vi "Limit_Line_Table.vi"() -> (0 "状态":string, 1 "Limit_ISL":string[][](array[string]), 2 "Limit_VSWR":string[][](array[string]), 3 "Limit_IL":string[][](array[string]))   [LabVIEW 2020]
uses:
  <vilib>/Utility/NIReport.llb/Report Type.ctl
  <vilib>/addons/_office/excel.llb/Excel Get Data ([str]).vi
  <vilib>/Utility/NIReport.llb/Append Text Table to Report (wrap).vi
  <vilib>/Utility/NIReport.llb/NI_report.lvclass
  <vilib>/Utility/NIReport.llb/NI_ReportGenerationCore.lvlib
  <vilib>/Utility/NIReport.llb/Excel/NI_Excel.lvclass
  <vilib>/addons/_office/NI_ReportGenerationToolkit.lvlib
panel:
  in  "插入损耗IL":i32(listbox)
  in  "驻波VSWR":i32(listbox) caption="多列列表框VSWR"
  in  "隔离度ISL":i32(listbox) caption="多列列表框VSWR"
  in  "清空":bool
  in  "导入":bool
  in  "保存":bool
  in  "取消":bool
  in  "确定":bool
  # "Limit Line"
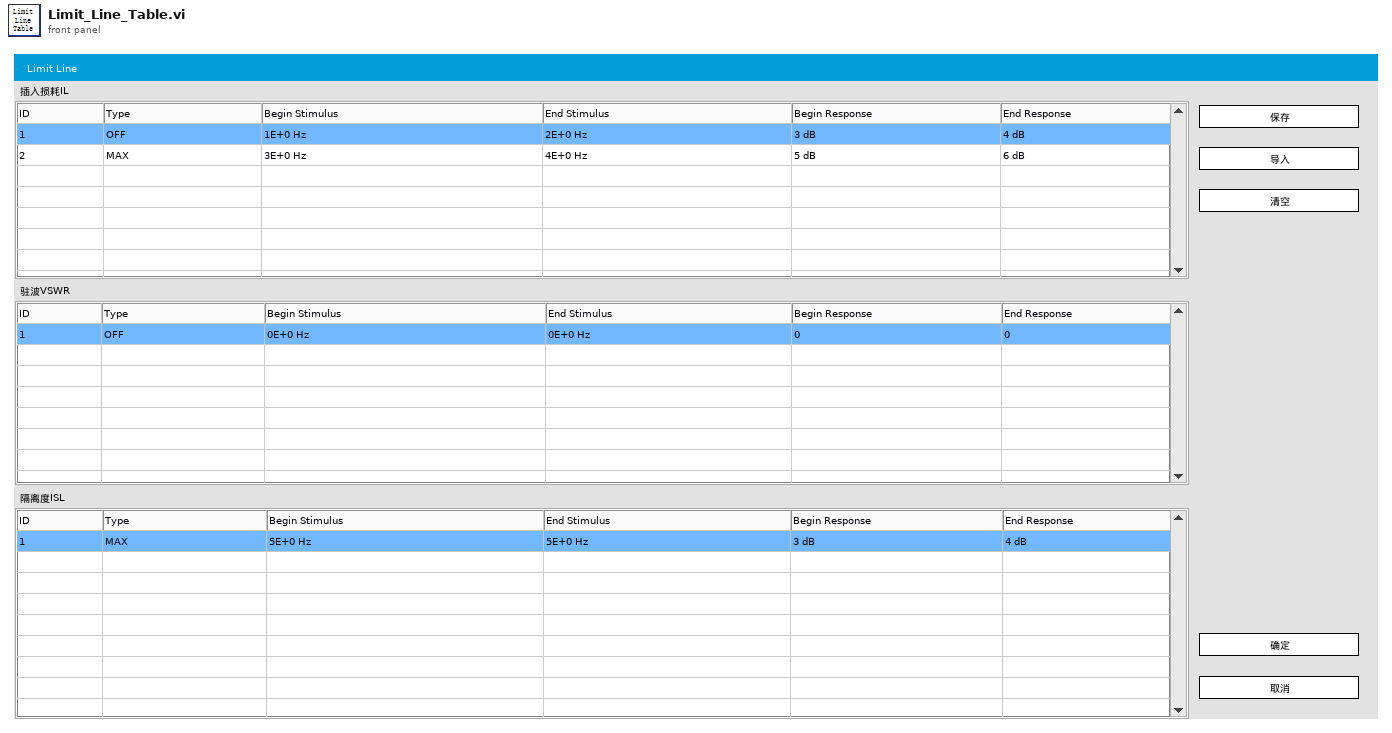
[diagram p1: front panel]
types:
  T1 = typedef "NI_ReportGenerationCore.lvlib/Report Type.ctl" = enum16{"HTML", "Word", "Excel"}
  T2 = enum16{"maximized", "minimized", "normal", "no change"}
  T3 = typedef "LVPoint32TypeDef.ctl" = cluster{"Horizontal":i32, "Vertical":i32}
  T4 = typedef "LVRowAndColumnTypeDef.ctl" = cluster{"Row":i32, "Column":i32}
  T5 = enum32{"invalid app kind", "Development System", "Run Time System", "Student Edition", "Embedded LabVIEW", "Evaluation", "Custom"}
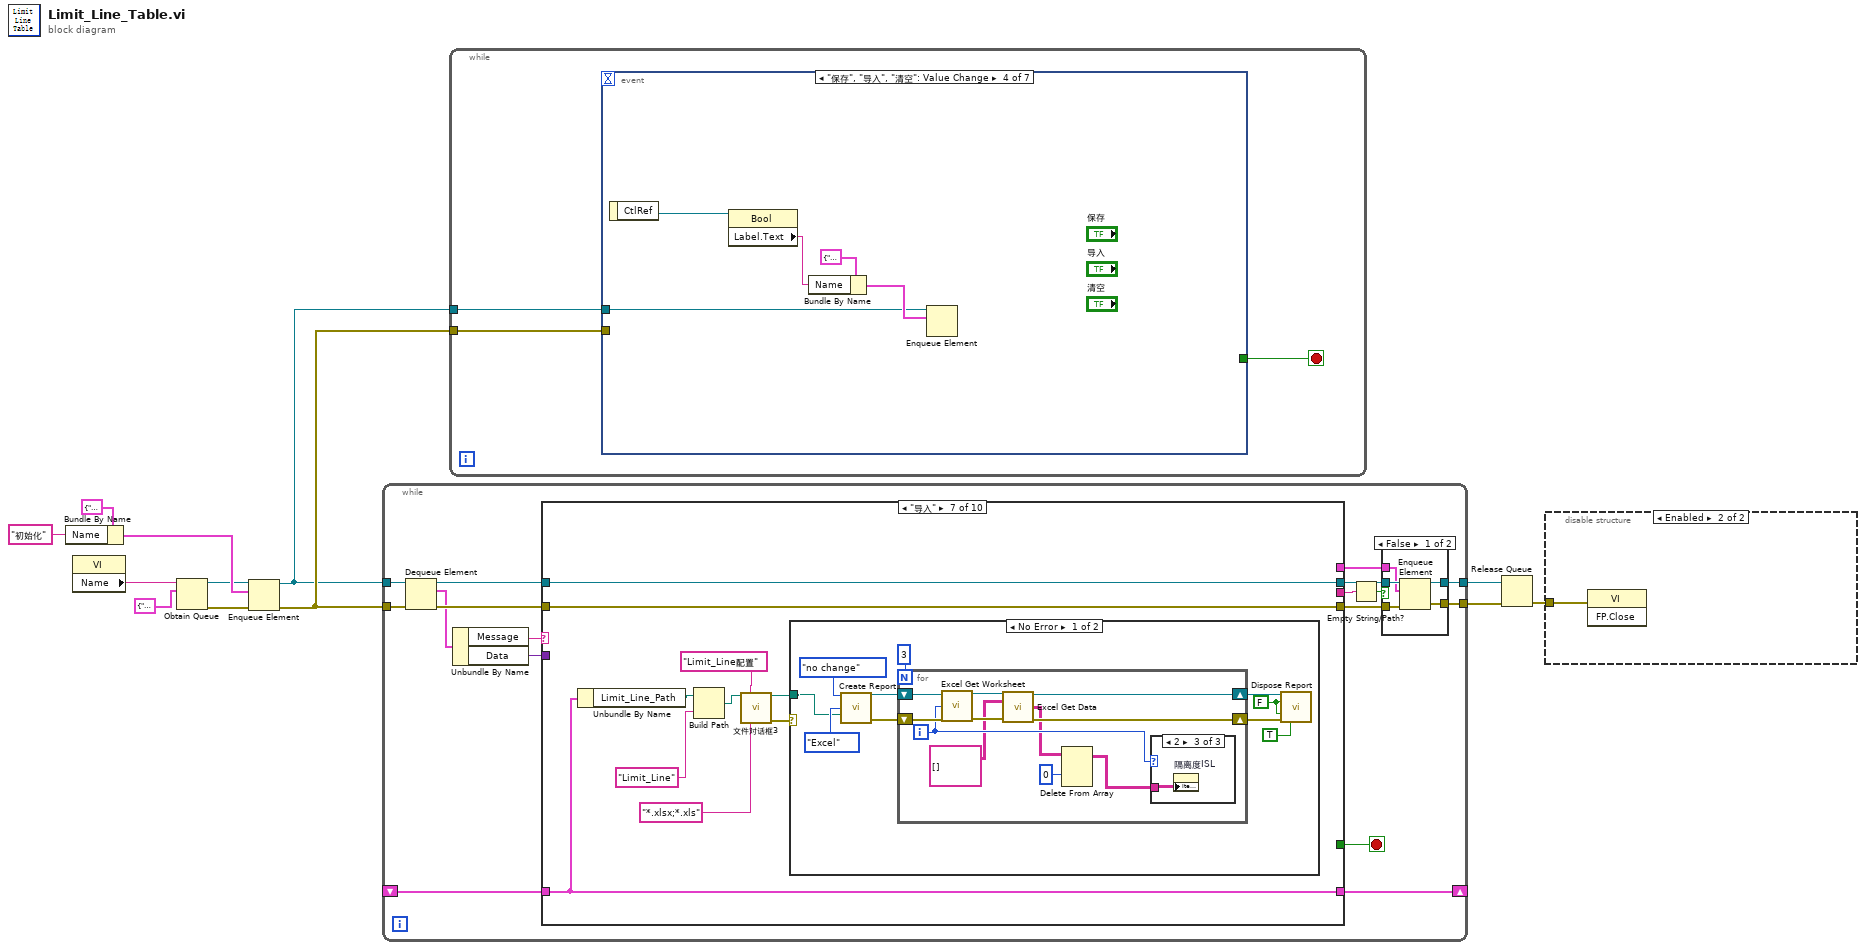
[diagram p0: block diagram]
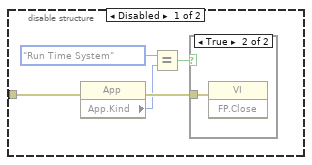
[diagram p2: hidden frame]
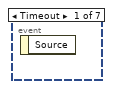
[diagram p4: hidden frame]
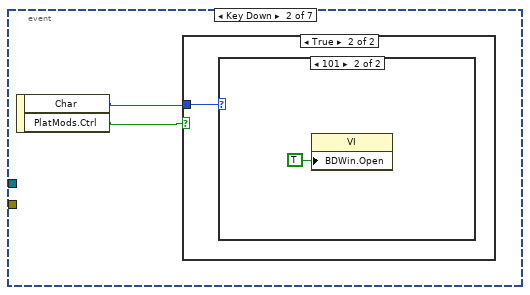
[diagram p5: hidden frame]
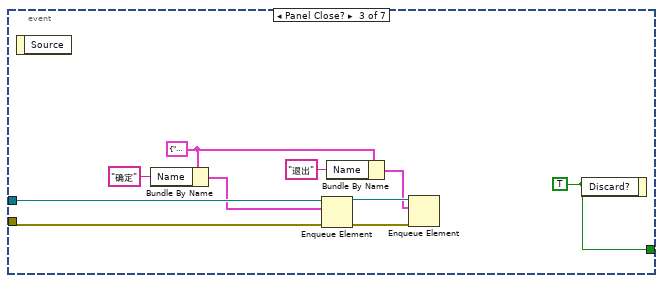
[diagram p8: hidden frame]
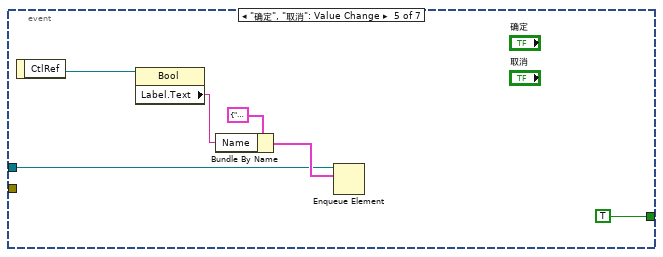
[diagram p9: hidden frame]
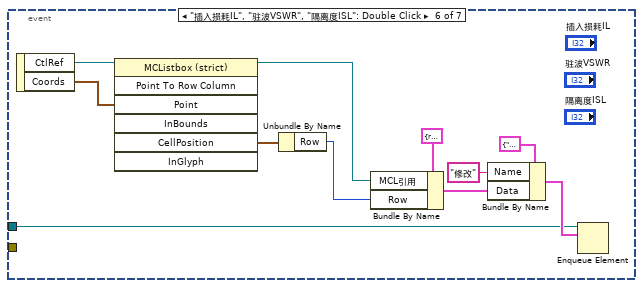
[diagram p10: hidden frame]
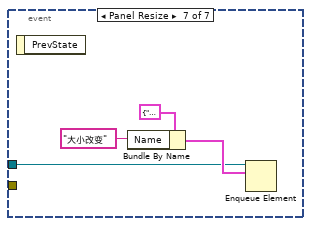
[diagram p11: hidden frame]
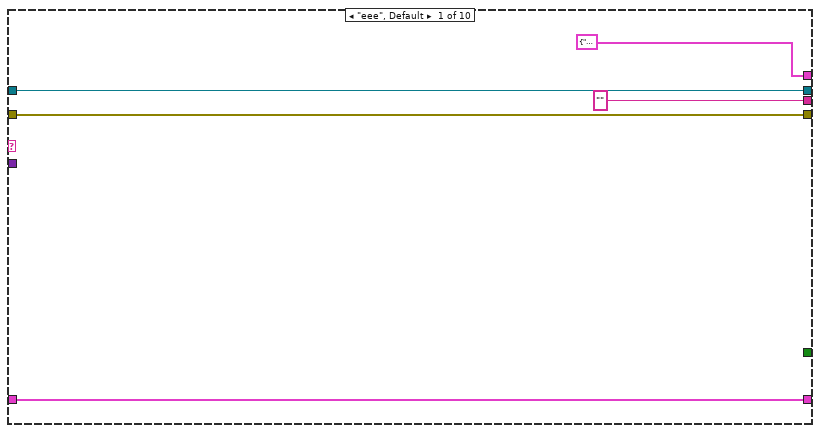
[diagram p13: hidden frame]
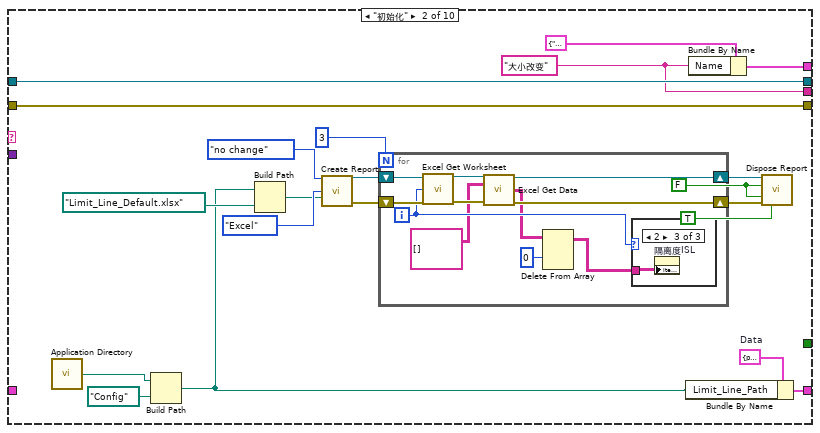
[diagram p14: hidden frame]
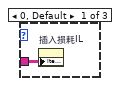
[diagram p15: hidden frame]
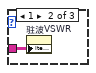
[diagram p16: hidden frame]
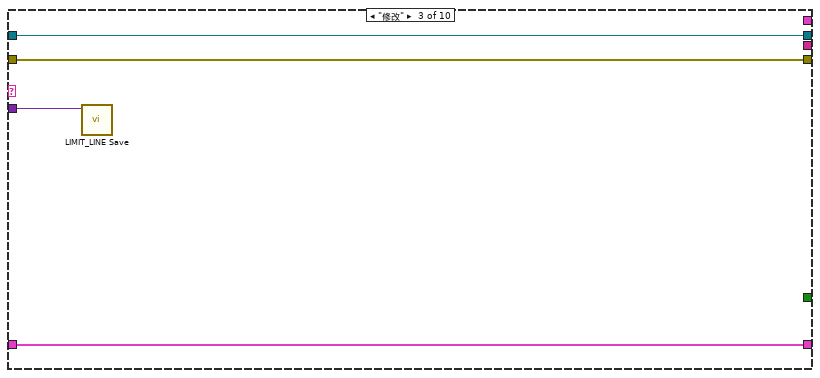
[diagram p17: hidden frame]
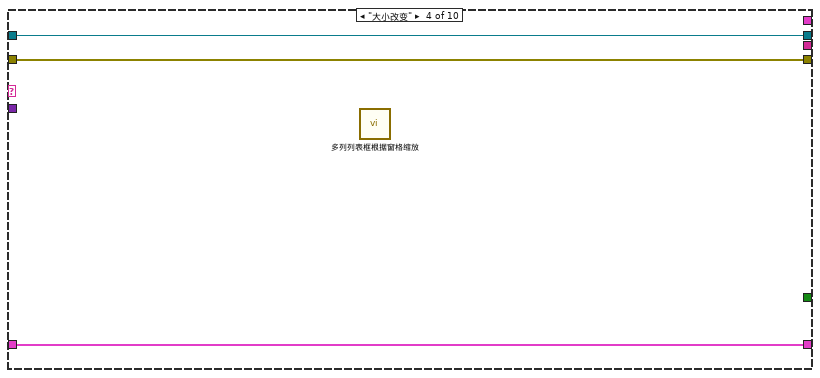
[diagram p18: hidden frame]
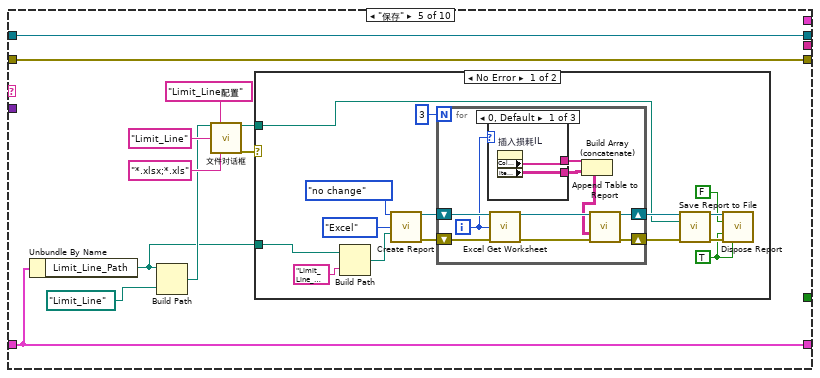
[diagram p19: hidden frame]
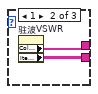
[diagram p20: hidden frame]
diagram:
  n1 = Bundle By Name(cluster=cluster{"Name":string, "Data":variant} {"Name"="", "Data"=variant}, "Name"="初始化") -> (w12:cluster{"Name":string, "Data":variant})
  n2 = property class="VI"() -> ("Name"=w2:string)  [unwired: 2 in, 2 out]
  n3 = Obtain Queue(name (unnamed)=w2, element data type=cluster{"Message":string, "Data":variant} {"Message"="", "Data"=variant}) -> (queue out=w4:refnum<queue>, error out=w3:errorcluster)  [unwired: 3 in, 1 out]
  n4 = Enqueue Element(queue=w4, element=w12, error in (no error)=w3) -> (queue out=w7:refnum<queue>, error out=w8:errorcluster)  [unwired: 1 in, 1 out]
  n5 = while {
    tunnel: w7 -> [w29]
    tunnel: w8 -> [w28]
    tunnel: [w23] -> w5
    tunnel: [w22] -> w6
    shift-right: [w14] -> _
    shift-left: _ -> [w13]
    stop <- w21 stop-if-true
    n6 = Dequeue Element(queue=w29, error in (no error)=w28) -> (queue out=w27:refnum<queue>, element=w17:cluster{"Message":string, "Data":variant}, error out=w24:errorcluster)  [unwired: 1 in, 1 out]
    n7 = Unbundle By Name(w17) -> ("Message"=w16:string, "Data"=w15:variant)
    n8 = case shown="\"导入\"" w16 {
      selector: w16 -> [_ _ _ _ _ _ _ w171 w211 _]
      tunnel: w27 -> [w41 w62 w80 w83 w94 w133 w145 w193 w217 w226]
      tunnel: [w41 w62 w80 w83 w94 w133 w145 w193 w217 w225] -> w26
      tunnel: [w40 w61 w79 w82 w93 w132 w144 w192 w216 w223] -> w25
      tunnel: w24 -> [w40 w61 w79 w82 w93 w132 w144 w192 w216 w224]
      tunnel: [_ _ _ _ _ _ _ _ _ TRUE] -> w21
      tunnel: ["" w57 _ _ _ _ _ w189 w213 _] -> w20
      tunnel: [cluster{"Name":string, "Data":variant} {"Name"="", "Data"=variant} w56 _ _ _ _ _ w190 w215 _] -> w18
      tunnel: w15 -> [_ _ w78 _ _ _ _ _ _ _]
      tunnel: [w37 w54 w77 w81 w87 w126 w142 w170 w210 w219] -> w14
      tunnel: w13 -> [w37 _ w77 w81 w87 w126 w142 w172 w212 w219]
      frame "eee", Default {
      }
      frame "初始化" {
        w48 = FALSE ("wait until printing completed? (T)")
        w55 = cluster{"Limit_Line_Path":path, "状态":string} {"Limit_Line_Path"=path "", "状态"=""}  # Data
        w57 = "大小改变"
        n9 = call <vilib>:"Application Directory.vi"() -> ("Application Directory"=w60:path)
        n10 = Build Path(base path=w60, name or relative path=path "Config" ("名称或相对路径")) -> (appended path=w42:path)
        n11 = Build Path(base path=w42, name or relative path=path "Limit_Line_Default.xlsx" ("名称或相对路径")) -> (appended path=w43:path)
        n12 = call <vilib>:"Create Report.vi"("window state (normal)"=T2."no change", "report type"=Report_Type."Excel", "template (empty)"=w43) -> ("report out"=w53:refnum<class "NI_report.lvclass">, "error out"=w52:errorcluster)  [unwired: 11 in]
        n13 = for {
          N: 3 -> [_]
          shift-right: [w68] -> w50
          shift-left: w53 -> [w71]
          shift-right: [w69] -> w51
          shift-left: w52 -> [w70]
          i -> [w67]
          n14 = call <vilib>:"Excel Get Worksheet.vi"("report in"=w71, "worksheet index (0)"=w67, "error in (no error)"=w70) -> ("report out"=w73:refnum<class "NI_report.lvclass">, "error out"=w72:errorcluster)  [unwired: 11 in]
          n15 = call-poly <vilib>:"Excel Get Data.vi"("report in"=w73, "data type"=string[][] [], "error in (no error)"=w72) -> ("report out"=w68:refnum<class "NI_report.lvclass">, "data"=w65:string[][], "error out"=w69:errorcluster)  [unwired: 10 in]
          n16 = Delete From Array(array=w65, index (row)=0) -> (array with subset deleted=w63:string[][])  [unwired: 2 in, 1 out]
          n17 = case shown="2" w67 {
            tunnel: w63 -> [w74 w75 w76]
            frame 0, Default {
              n18 = property on="插入损耗IL" class="MCListbox (strict)"("ItemNames"=w74) -> ()  [unwired: 2 in, 2 out]
            }
            frame 1 {
              n19 = property on="驻波VSWR" class="MCListbox (strict)"("ItemNames"=w75) -> ()  [unwired: 2 in, 2 out]
            }
            frame 2 {
              n20 = property on="隔离度ISL" class="MCListbox (strict)"("ItemNames"=w76) -> ()  [unwired: 2 in, 2 out]
            }
          }
        }
        n21 = Bundle By Name(cluster=w55, "Limit_Line_Path"=w42) -> (w54:cluster{"Limit_Line_Path":path, "状态":string})
        n22 = Bundle By Name(cluster=cluster{"Name":string, "Data":variant} {"Name"="", "Data"=variant}, "Name"=w57) -> (w56:cluster{"Name":string, "Data":variant})
        n23 = call-dynamic "Dispose Report.vi"("report in"=w50, "wait until printing completed? (T)"=w48, "save changes? (F)"=w48, "error in (no error)"=w51, "close report? (T)"=TRUE ("wait until printing completed? (T)")) -> ()  [unwired: 10 in, 1 out]
      }
      frame "修改" {
        n24 = call "LIMIT_LINE Save.vi"("data"=w78) -> ()  [unwired: 11 in]
      }
      frame "大小改变" {
        n25 = call "多列列表框根据窗格缩放.vi"() -> ()  [unwired: 11 in, 1 out]
      }
      frame "保存" {
        n26 = Unbundle By Name(w87) -> ("Limit_Line_Path"=w84:path)
        n27 = Build Path(base path=w84, name or relative path=path "Limit_Line") -> (appended path=w85:path)
        n28 = call "文件对话框"("start path"=w85, "prompt"="Limit_Line配置" ("default name"), "default name"="Limit_Line", "pattern (all files)"="*.xlsx;*.xls") -> ("selected path"=w92:path, "error out"=w91:errorcluster)  [unwired: 8 in, 2 out]
        n29 = case shown="No Error" w91 {
          tunnel: w92 -> [w98 _]
          tunnel: w84 -> [w95 _]
          frame No Error {
            w103 = TRUE ("save changes? (F)")
            n30 = Build Path(base path=w95, name or relative path="Limit_Line_Template.xlsx") -> (appended path=w96:path)
            n31 = call <vilib>:"Create Report.vi"("window state (normal)"=T2."no change", "report type"=Report_Type."Excel", "template (empty)"=w96) -> ("report out"=w100:refnum<class "NI_report.lvclass">, "error out"=w101:errorcluster)  [unwired: 11 in]
            n32 = for {
              N: 3 -> [_]
              shift-right: [w118] -> w107
              shift-left: w101 -> [w117]
              shift-right: [w119] -> w108
              shift-left: w100 -> [w115]
              i -> [w111]
              n33 = case shown="0, Default" w111 {
                tunnel: [w121 w123 w125] -> w112
                tunnel: [w120 w122 w124] -> w113
                frame 0, Default {
                  n34 = property on="插入损耗IL" class="MCListbox (strict)"() -> ("ColHdrString"=w121:string[], "ItemNames"=w120:string[][])  [unwired: 2 in, 2 out]
                }
                frame 1 {
                  n35 = property on="驻波VSWR" class="MCListbox (strict)"() -> ("ColHdrString"=w123:string[], "ItemNames"=w122:string[][])  [unwired: 2 in, 2 out]
                }
                frame 2 {
                  n36 = property on="隔离度ISL" class="MCListbox (strict)"() -> ("ColHdrString"=w125:string[], "ItemNames"=w124:string[][])  [unwired: 2 in, 2 out]
                }
              }
              n37 = call <vilib>:"Excel Get Worksheet.vi"("report in"=w115, "worksheet index (0)"=w111, "error in (no error)"=w117) -> ("report out"=w114:refnum<class "NI_report.lvclass">, "error out"=w116:errorcluster)  [unwired: 11 in]
              n38 = Build Array (concatenate)(w112, w113) -> (w110:string[][])
              n39 = call-poly <vilib>:"Append Table to Report.vi"("report in"=w114, "text data"=w110, "error in (no error)"=w116) -> ("report out"=w119:refnum<class "NI_report.lvclass">, "error out"=w118:errorcluster)  [unwired: 9 in, 2 out]
            }
            n40 = call-dynamic "Save Report to File.vi"("report in"=w108, "report file path"=w98, "error in (no error)"=w107) -> ("report out"=w106:refnum<class "NI_report.lvclass">, "error out"=w105:errorcluster)  [unwired: 11 in]
            n41 = call-dynamic "Dispose Report.vi"("report in"=w106, "wait until printing completed? (T)"=FALSE, "save changes? (F)"=w103, "error in (no error)"=w105, "close report? (T)"=w103) -> ()  [unwired: 10 in, 1 out]
          }
          frame Error {
          }
        }
      }
      frame "清空" {
        n42 = control-ref of="插入损耗IL"() -> (w131:refnum<vi>)
        n43 = control-ref of="驻波VSWR"() -> (w130:refnum<vi>)
        n44 = control-ref of="隔离度ISL"() -> (w129:refnum<vi>)
        n45 = Build Array(w131, w130, w129) -> (w128:refnum<vi>[])
        n46 = for {
          tunnel: w128 -> [w135] mode=indexing
          tunnel: string[][] [] ("项名") -> [w134]
          n47 = property class="MCListbox (strict)"(reference=w135, "ItemNames"=w134) -> ()  [unwired: 1 in, 2 out]
        }
      }
      frame "导入" {
        n48 = Unbundle By Name(w142) -> ("Limit_Line_Path"=w138:path)
        n49 = Build Path(base path=w138, name or relative path="Limit_Line" ("default name")) -> (appended path=w136:path)
        n50 = call "文件对话框3"("start path"=w136, "prompt"="Limit_Line配置" ("default name"), "pattern (all files)"="*.xlsx;*.xls") -> ("selected path"=w139:path, "error out"=w140:errorcluster)  [unwired: 9 in, 2 out]
        n51 = case shown="No Error" w140 {
          tunnel: w139 -> [w154 _]
          frame No Error {
            w147 = FALSE ("wait until printing completed? (T)")
            n52 = call <vilib>:"Create Report.vi"("window state (normal)"=T2."no change", "report type"=Report_Type."Excel", "template (empty)"=w154) -> ("report out"=w152:refnum<class "NI_report.lvclass">, "error out"=w151:errorcluster)  [unwired: 11 in]
            n53 = for {
              N: 3 -> [_]
              shift-right: [w161] -> w149
              shift-left: w152 -> [w164]
              shift-right: [w162] -> w150
              shift-left: w151 -> [w163]
              i -> [w160]
              n54 = call <vilib>:"Excel Get Worksheet.vi"("report in"=w164, "worksheet index (0)"=w160, "error in (no error)"=w163) -> ("report out"=w166:refnum<class "NI_report.lvclass">, "error out"=w165:errorcluster)  [unwired: 11 in]
              n55 = call-poly <vilib>:"Excel Get Data.vi"("report in"=w166, "data type"=string[][] [], "error in (no error)"=w165) -> ("report out"=w161:refnum<class "NI_report.lvclass">, "data"=w158:string[][], "error out"=w162:errorcluster)  [unwired: 10 in]
              n56 = Delete From Array(array=w158, index (row)=0) -> (array with subset deleted=w156:string[][])  [unwired: 2 in, 1 out]
              n57 = case shown="2" w160 {
                tunnel: w156 -> [w167 w168 w169]
                frame 0, Default {
                  n58 = property on="插入损耗IL" class="MCListbox (strict)"("ItemNames"=w167) -> ()  [unwired: 2 in, 2 out]
                }
                frame 1 {
                  n59 = property on="驻波VSWR" class="MCListbox (strict)"("ItemNames"=w168) -> ()  [unwired: 2 in, 2 out]
                }
                frame 2 {
                  n60 = property on="隔离度ISL" class="MCListbox (strict)"("ItemNames"=w169) -> ()  [unwired: 2 in, 2 out]
                }
              }
            }
            n61 = call-dynamic "Dispose Report.vi"("report in"=w149, "wait until printing completed? (T)"=w147, "save changes? (F)"=w147, "error in (no error)"=w150, "close report? (T)"=TRUE ("wait until printing completed? (T)")) -> ()  [unwired: 10 in, 1 out]
          }
          frame Error {
          }
        }
      }
      frame "确定" {
        w177 = TRUE ("save changes? (F)")
        w189 = "退出" ("Name")
        n62 = Bundle By Name(cluster=w172, "状态"=w171) -> (w170:cluster{"Limit_Line_Path":path, "状态":string})
        n63 = Unbundle By Name(w170) -> ("Limit_Line_Path"=w173:path)
        n64 = Build Path(base path=w173, name or relative path="Limit_Line_Template.xlsx") -> (appended path=w181:path)
        n65 = call <vilib>:"Create Report.vi"("window state (normal)"=T2."no change", "report type"=Report_Type."Excel", "template (empty)"=w181) -> ("report out"=w182:refnum<class "NI_report.lvclass">, "error out"=w183:errorcluster)  [unwired: 11 in]
        n66 = for {
          N: 3 -> [_]
          shift-right: [w202] -> w186
          shift-left: w183 -> [w201]
          shift-right: [w203] -> w187
          shift-left: w182 -> [w199]
          i -> [w195]
          n67 = case shown="0, Default" w195 {
            tunnel: [w205 w207 w209] -> w196
            tunnel: [w204 w206 w208] -> w197
            frame 0, Default {
              n68 = property on="插入损耗IL" class="MCListbox (strict)"() -> ("ColHdrString"=w205:string[], "ItemNames"=w204:string[][])  [unwired: 2 in, 2 out]
            }
            frame 1 {
              n69 = property on="驻波VSWR" class="MCListbox (strict)"() -> ("ColHdrString"=w207:string[], "ItemNames"=w206:string[][])  [unwired: 2 in, 2 out]
            }
            frame 2 {
              n70 = property on="隔离度ISL" class="MCListbox (strict)"() -> ("ColHdrString"=w209:string[], "ItemNames"=w208:string[][])  [unwired: 2 in, 2 out]
            }
          }
          n71 = call <vilib>:"Excel Get Worksheet.vi"("report in"=w199, "worksheet index (0)"=w195, "error in (no error)"=w201) -> ("report out"=w198:refnum<class "NI_report.lvclass">, "error out"=w200:errorcluster)  [unwired: 11 in]
          n72 = Build Array (concatenate)(w196, w197) -> (w194:string[][])
          n73 = call-poly <vilib>:"Append Table to Report.vi"("report in"=w198, "text data"=w194, "error in (no error)"=w200) -> ("report out"=w203:refnum<class "NI_report.lvclass">, "error out"=w202:errorcluster)  [unwired: 9 in, 2 out]
        }
        n74 = Build Path(base path=w173, name or relative path=path "Limit_Line_Default.xlsx" ("名称或相对路径")) -> (appended path=w174:path)
        n75 = Bundle By Name(cluster=cluster{"Name":string, "Data":variant} {"Name"="", "Data"=variant}, "Name"=w189) -> (w190:cluster{"Name":string, "Data":variant})
        n76 = call-dynamic "Save Report to File.vi"("report in"=w187, "report file path"=w174, "error in (no error)"=w186) -> ("report out"=w185:refnum<class "NI_report.lvclass">, "error out"=w184:errorcluster)  [unwired: 11 in]
        n77 = call-dynamic "Dispose Report.vi"("report in"=w185, "wait until printing completed? (T)"=FALSE, "save changes? (F)"=w177, "error in (no error)"=w184, "close report? (T)"=w177) -> ()  [unwired: 10 in, 1 out]
      }
      frame "取消" {
        w213 = "退出" ("Name")
        n78 = Bundle By Name(cluster=w212, "状态"=w211) -> (w210:cluster{"Limit_Line_Path":path, "状态":string})
        n79 = Bundle By Name(cluster=cluster{"Name":string, "Data":variant} {"Name"="", "Data"=variant}, "Name"=w213) -> (w215:cluster{"Name":string, "Data":variant})
      }
      frame "退出" {
        n80 = property on="插入损耗IL" class="MulticolumnListbox (strict)"() -> ("ItemNames"=→"Limit_IL":string[][])  [unwired: 2 in, 2 out]
        n81 = property on="驻波VSWR" class="MulticolumnListbox (strict)"() -> ("ItemNames"=→"Limit_VSWR":string[][])  [unwired: 2 in, 2 out]
        n82 = property on="隔离度ISL" class="MulticolumnListbox (strict)"() -> ("ItemNames"=→"Limit_ISL":string[][])  [unwired: 2 in, 2 out]
        n83 = Unbundle By Name(w219) -> ("状态"=→"状态":string)
        n84 = Flush Queue(queue=w226, error in (no error)=w224) -> (queue out=w225:refnum<queue>, error out=w223:errorcluster)  [unwired: 1 out]
      }
    }
    n85 = Empty String/Path?(string/path=w20) -> (empty?=w19:bool)
    n86 = case shown="False" w19 {
      tunnel: w26 -> [w34 w36]
      tunnel: w25 -> [w33 w35]
      tunnel: [w32 w35] -> w23
      tunnel: [w31 w36] -> w22
      tunnel: w18 -> [w30 _]
      frame False {
        n87 = Enqueue Element(queue=w34, element=w30, error in (no error)=w33) -> (queue out=w31:refnum<queue>, error out=w32:errorcluster)  [unwired: 1 in, 1 out]
      }
      frame True {
      }
    }
  }
  n88 = while {
    tunnel: w7 -> [w229]
    tunnel: w8 -> [w228]
    stop <- w230 stop-if-true
    n89 = event shown="[3] \"保存\", \"导入\", \"清空\": Value Change" {
      selector: _ -> [_ _ _ _ _ _ _]
      dyn-events: _ -> [_ _ _ _ _ _ _]
      timeout: _ -> [_ _ _ _ _ _ _]
      tunnel: [_ _ w244 _ TRUE ("放弃？") _ _] -> w230
      tunnel: w229 -> [_ _ w242 w246 w252 w260 w268]
      tunnel: w228 -> [_ _ w243 _ _ _ _]
      event Timeout {
        n90 = event-data() -> ()  [unwired: 1 in, 1 out]
      }
      event Key Down {
        n91 = event-data() -> ("Char"=w232:i16, "PlatMods.Ctrl"=w231:bool)  [unwired: 1 in]
        n92 = case shown="True" w231 {
          tunnel: w232 -> [_ w233]
          frame False {
          }
          frame True {
            n93 = case shown="101" w233 {
              frame 0, Default {
              }
              frame 101 {
                n94 = property class="VI"("BDWin.Open"=TRUE ("程序框图窗口:打开")) -> ()  [unwired: 2 in, 2 out]
              }
            }
          }
        }
      }
      event Panel Close? {
        w237 = cluster{"Name":string, "Data":variant} {"Name"="", "Data"=variant}
        w244 = TRUE ("放弃？")
        n95 = event-data() -> ()  [unwired: 1 in, 1 out]
        n96 = Bundle By Name(cluster=w237, "Name"="确定" ("元素")) -> (w238:cluster{"Name":string, "Data":variant})
        n97 = Enqueue Element(queue=w242, element=w238, error in (no error)=w243) -> (queue out=w240:refnum<queue>, error out=w239:errorcluster)  [unwired: 1 in, 1 out]
        n98 = Bundle By Name(cluster=w237, "Name"="退出") -> (w236:cluster{"Name":string, "Data":variant})
        n99 = Enqueue Element(queue=w240, element=w236, error in (no error)=w239) -> ()  [unwired: 1 in, 3 out]
        n100 = event-data("Discard?"=w244) -> ()  [unwired: 1 in, 1 out]
      }
      event "保存", "导入", "清空": Value Change {
        n101 = event-data() -> ("CtlRef"=w249:refnum<vi>)  [unwired: 1 in]
        n102 = property class="Bool"(reference=w249) -> ("Label.Text"=w245:string)  [unwired: 1 in, 2 out]
        n103 = Bundle By Name(cluster=cluster{"Name":string, "Data":variant} {"Name"="", "Data"=variant}, "Name"=w245) -> (w248:cluster{"Name":string, "Data":variant})
        n104 = Enqueue Element(queue=w246, element=w248) -> ()  [unwired: 2 in, 3 out]
      }
      event "确定", "取消": Value Change {
        n105 = event-data() -> ("CtlRef"=w255:refnum<vi>)  [unwired: 1 in]
        n106 = property class="Bool"(reference=w255) -> ("Label.Text"=w251:string)  [unwired: 1 in, 2 out]
        n107 = Bundle By Name(cluster=cluster{"Name":string, "Data":variant} {"Name"="", "Data"=variant}, "Name"=w251) -> (w254:cluster{"Name":string, "Data":variant})
        n108 = Enqueue Element(queue=w252, element=w254) -> ()  [unwired: 2 in, 3 out]
      }
      event "插入损耗IL", "驻波VSWR", "隔离度ISL": Double Click {
        n109 = event-data() -> ("CtlRef"=w265:refnum<vi>, "Coords"=w264:T3)  [unwired: 1 in]
        n110 = invoke class="MCListbox (strict)" method="Point To Row Column"(reference=w265, "Point"=w264) -> (reference out=w258:refnum<vi>, "CellPosition"=w266:T4)  [unwired: 5 in, 5 out]
        n111 = Unbundle By Name(w266) -> ("Row"=w256:i32)
        n112 = Bundle By Name(cluster=cluster{"MCL引用":refnum<vi>, "Row":i32} {"MCL引用"=refnum, "Row"=0}, "MCL引用"=w258, "Row"=w256) -> (w257:cluster{"MCL引用":refnum<vi>, "Row":i32})
        n113 = Bundle By Name(cluster=cluster{"Name":string, "Data":variant} {"Name"="", "Data"=variant}, "Name"="修改" ("message"), "Data"=w257) -> (w263:cluster{"Name":string, "Data":variant})
        n114 = Enqueue Element(queue=w260, element=w263) -> ()  [unwired: 2 in, 3 out]
      }
      event Panel Resize {
        n115 = event-data() -> ()  [unwired: 1 in, 1 out]
        n116 = Bundle By Name(cluster=cluster{"Name":string, "Data":variant} {"Name"="", "Data"=variant}, "Name"="大小改变" ("message")) -> (w270:cluster{"Name":string, "Data":variant})
        n117 = Enqueue Element(queue=w268, element=w270) -> ()  [unwired: 2 in, 3 out]
      }
    }
  }
  n118 = Release Queue(queue=w6, error in (no error)=w5) -> (error out=w1:errorcluster)  [unwired: 1 in, 2 out]
  n119 = disable-structure shown="Enabled" {
    disable-tunnel: w1 -> [w271 w277]
    frame Disabled {
      n120 = property class="App"(error in=w271) -> (error out=w274:errorcluster, "App.Kind"=w272:T5)  [unwired: 1 in, 1 out]
      n121 = Equal?(x=T5."Run Time System" ("y"), y=w272) -> (x = y?=w275:bool)
      n122 = case shown="True" w275 {
        tunnel: w274 -> [_ w276]
        frame False {
        }
        frame True {
          n123 = invoke class="VI" method="FP.Close"(error in=w276) -> ()  [unwired: 2 in, 3 out]
        }
      }
    }
    frame Enabled {
      n124 = invoke class="VI" method="FP.Close"(error in=w277) -> ()  [unwired: 2 in, 3 out]
    }
  }
